vi "Read_LogFiles (Host Computer).vi"() -> ()   [LabVIEW 2017]
uses:
  <vilib>/Utility/file.llb/Read From Spreadsheet File (DBL).vi
panel:
  out "Graph 3":cluster{dbl[], dbl[]}(graph)
  out "Graph 2":cluster{"Y":dbl[], "Y":dbl[]}[](graph)
  out "Graph 1":cluster{"Y":dbl[], "Y":dbl[]}[](graph)
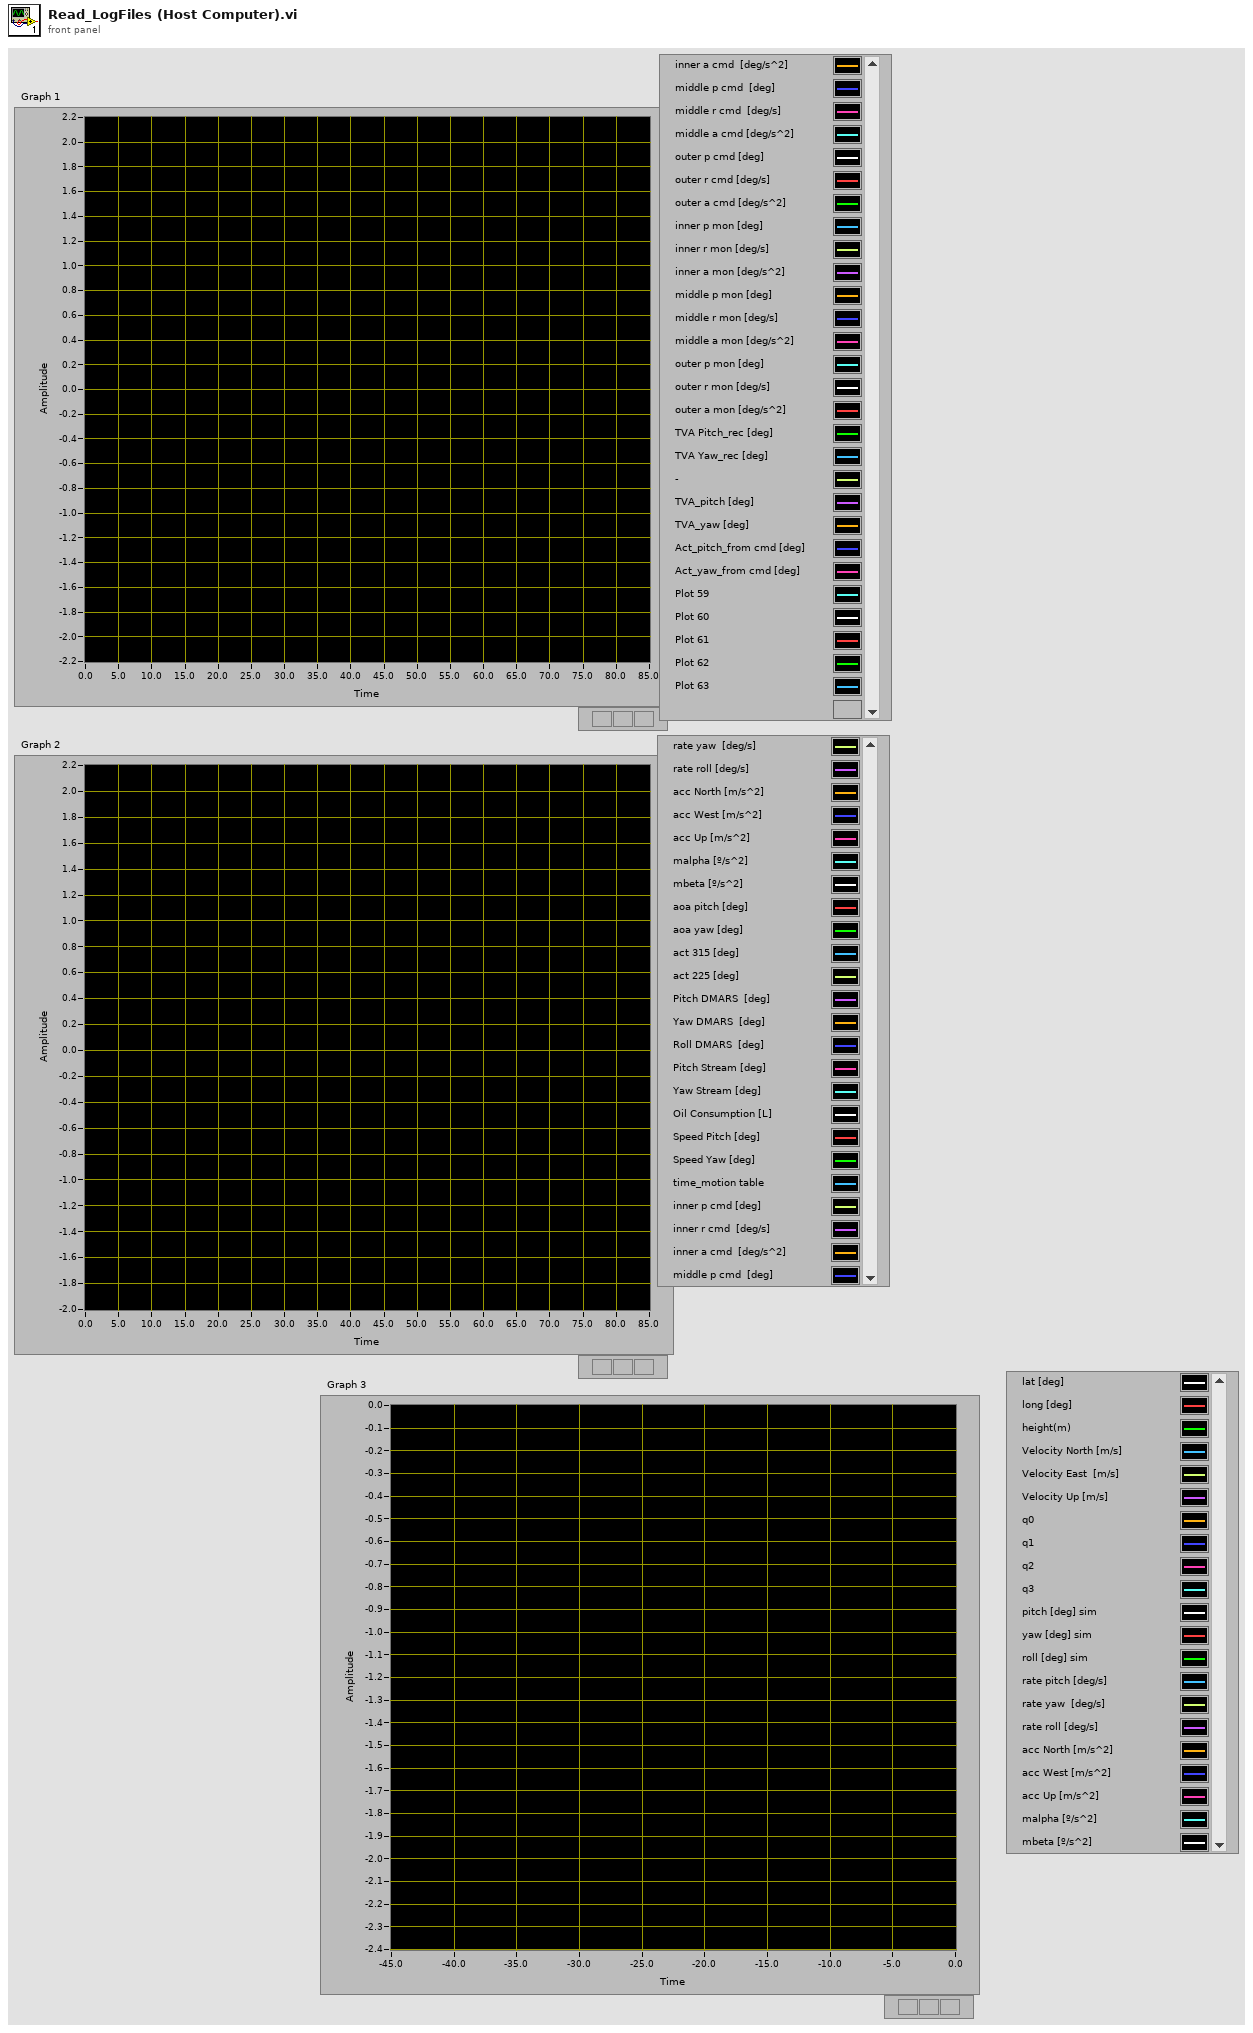
[diagram p1: front panel]
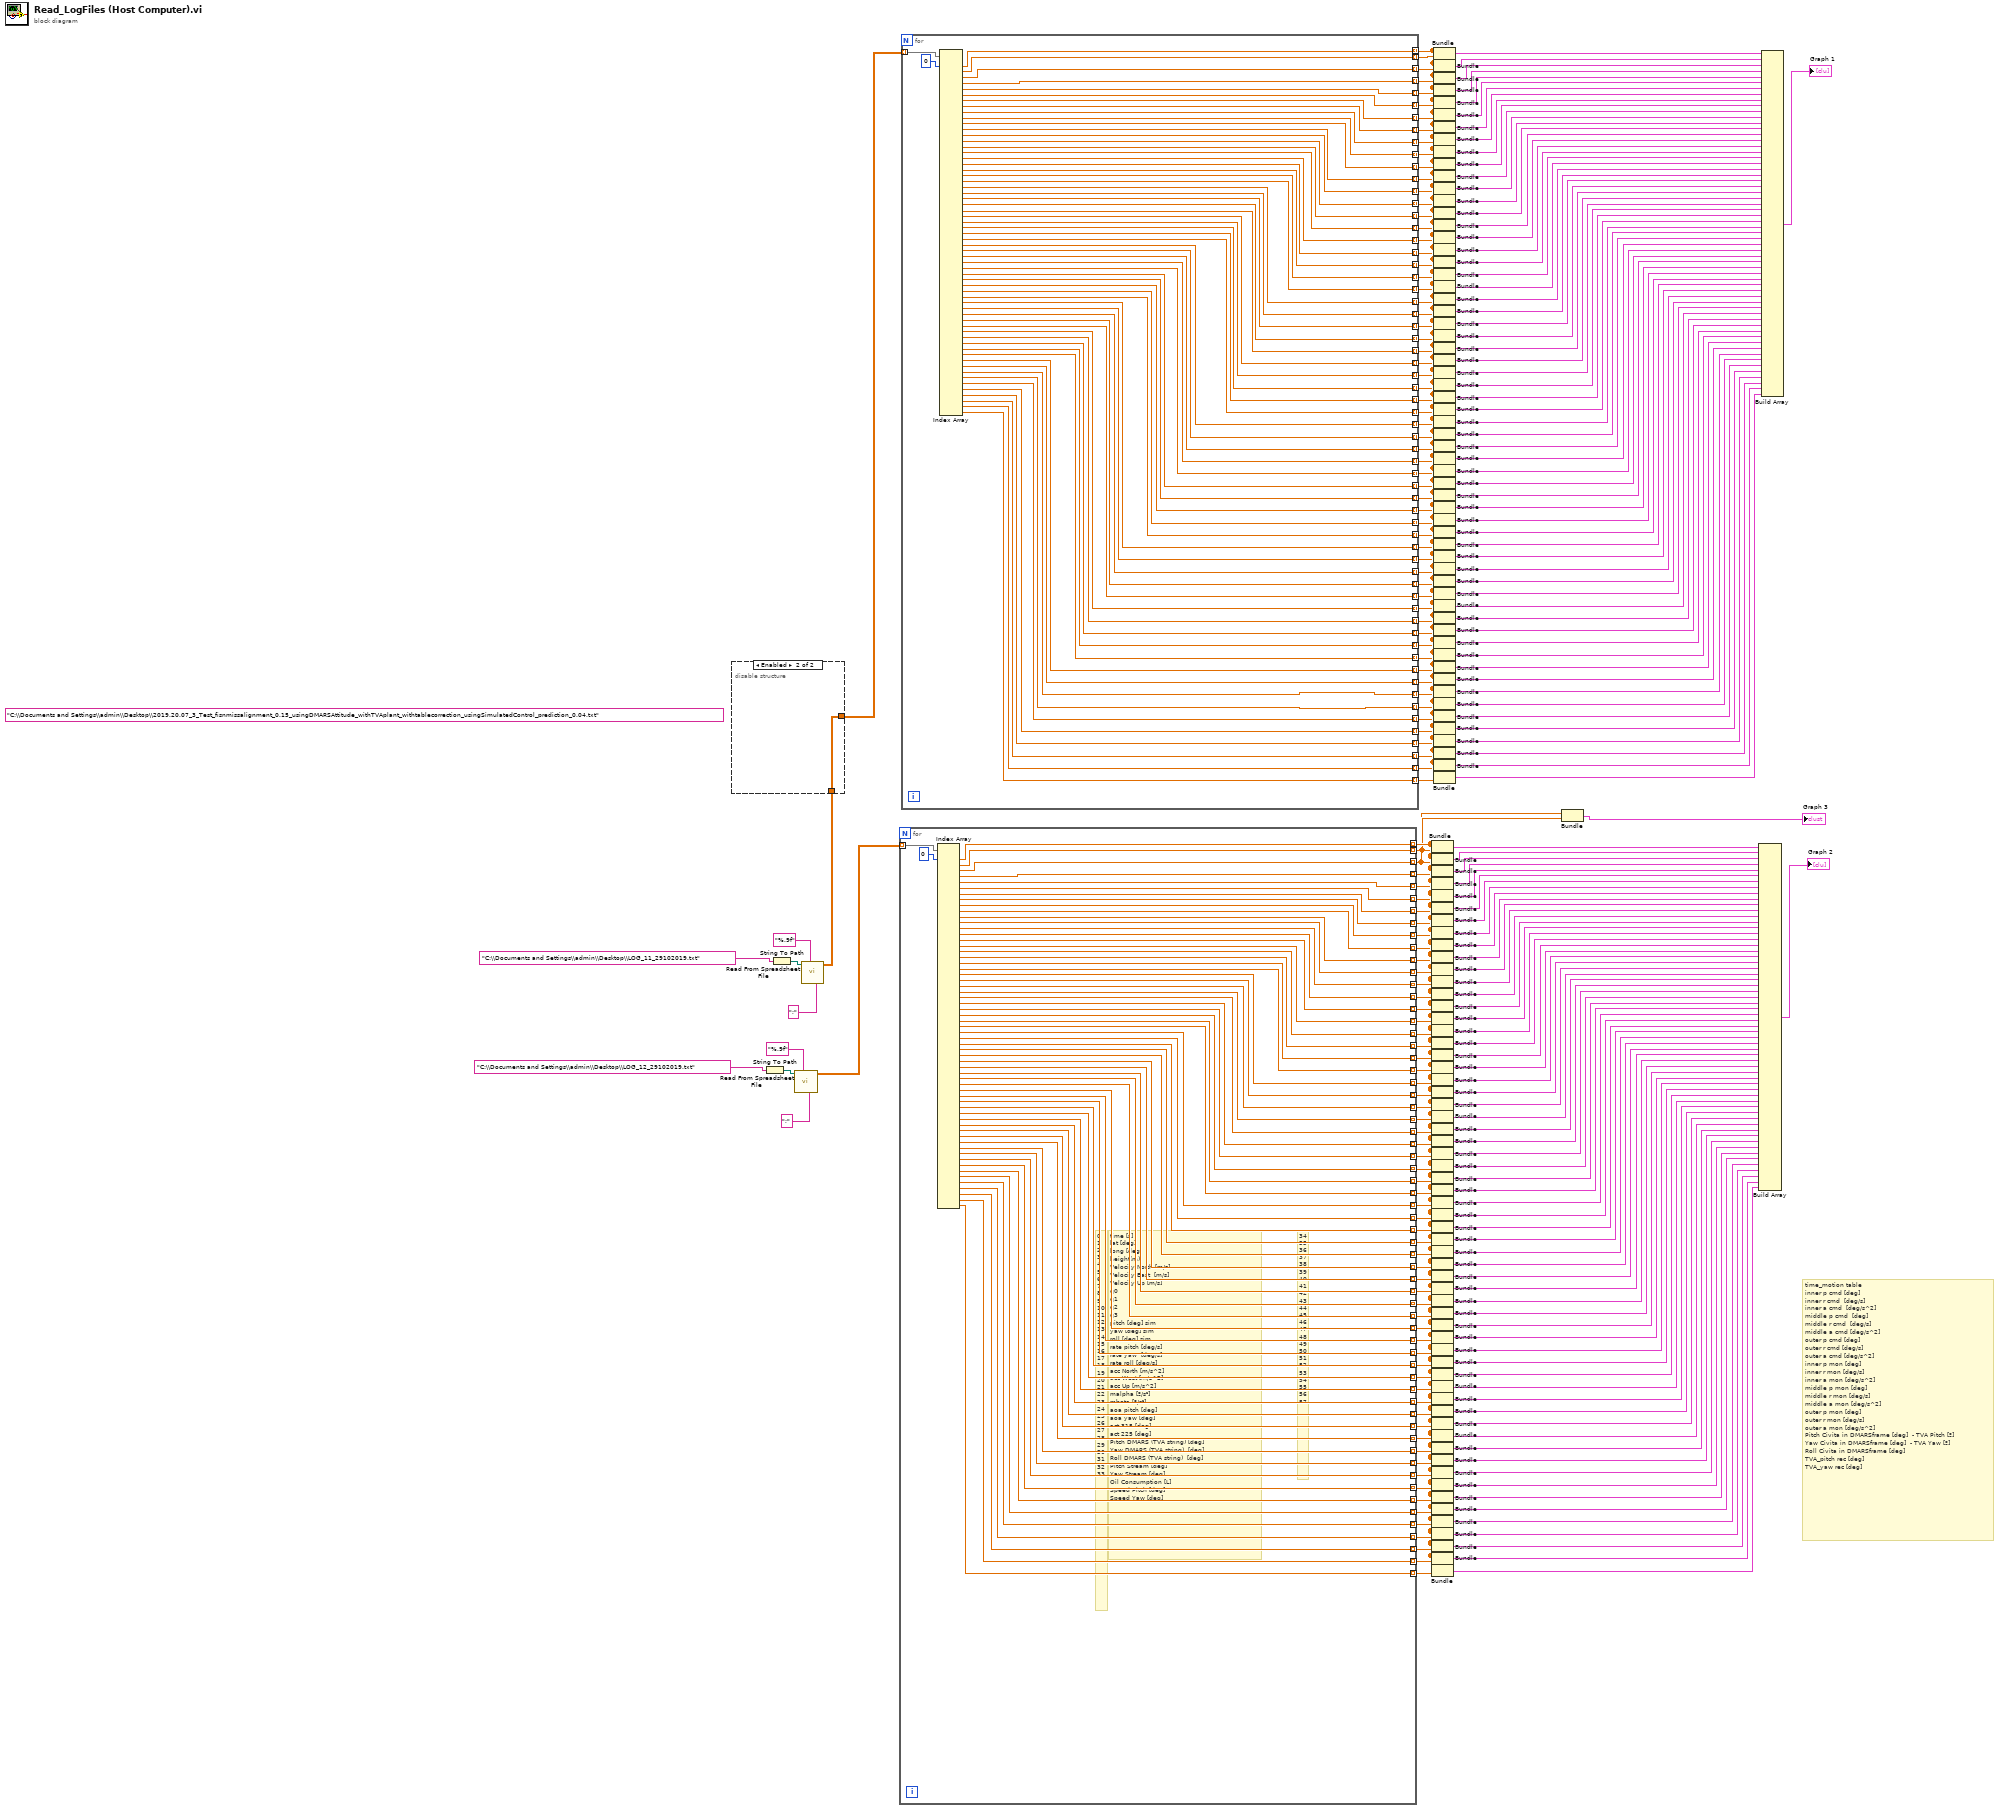
[diagram p0: block diagram]
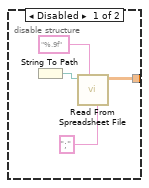
[diagram p2: hidden frame]
diagram:
  (unwired) "C:\\Documents and Settings\\admin\\Desktop\\2019.20.07_3_Test_fisnmissalignment_0.15_usingDMARSAttitude_withTVAplant_withtablecorrection_usingSimulatedControl_prediction_0.04.txt" ("format (%.3f)")
  # "time_motion table\ninner p cmd [deg]\ninner r cmd  [deg/s]\ninner a cmd  [deg/s^2]\nmiddle p cmd  [deg]\nmiddle r cmd  [deg/s]\nmiddle a cmd [deg/s^2]\nouter p cmd [deg]\nouter r cmd [deg/s]\nouter a cmd [deg/s^2]\ninner p mon [deg]\ninner r mon [deg/s]\ninner a mon [deg/s^2]\nmiddle p mon [deg]\nmiddle r mon [deg/s]\nmiddle a mon [deg/s^2]\nouter p mon [deg]\nouter r mon [deg/s]\nouter a mon [deg/s^2]\nPitch Civita in DMARSframe [deg]  - TVA Pitch [º]\nYaw Civita in DMARSframe [deg]  - TVA Yaw [º]\nRoll Civita in DMARSframe [deg]\nTVA_pitch rec [deg]\nTVA_yaw rec [deg]"
  # "34\n35\n36\n37\n38\n39\n40\n41\n42\n43\n44\n45\n46\n47\n48\n49\n50\n51\n52\n53\n54\n55\n56\n57"
  # "0\n1\n2\n3\n4\n5\n6\n7\n8\n9\n10\n11\n12\n13\n14\n15\n16\n17\n18\n19\n20\n21\n22\n23\n24\n25\n26\n27\n28\n29\n30\n31\n32\n33"
  # "time [s]\nlat [deg]\nlong [deg]\nheight(m)\nVelocity North [m/s]\nVelocity East  [m/s]\nVelocity Up [m/s]\nq0\nq1\nq2\nq3\npitch [deg] sim\nyaw [deg] sim\nroll [deg] sim\nrate pitch [deg/s] \nrate yaw  [deg/s]\nrate roll [deg/s]\nacc North [m/s^2] \nacc West [m/s^2]\nacc Up [m/s^2]\nmalpha [º/s²]\nmbeta [º/s²]\naoa pitch [deg] \naoa yaw [deg]\nact 315 [deg] \nact 225 [deg]\nPitch DMARS (TVA string) [deg]\nYaw DMARS (TVA string)  [deg]\nRoll DMARS (TVA string)  [deg]\nPitch Stream [deg]\nYaw Stream [deg]\nOil Consumption [L]\nSpeed Pitch [deg]\nSpeed Yaw [deg]"
  n1 = String To Path(string="C:\\Documents and Settings\\admin\\Desktop\\LOG_12_29102019.txt" ("format (%.3f)")) -> (path=w127:path)
  n2 = String To Path(string="C:\\Documents and Settings\\admin\\Desktop\\LOG_11_29102019.txt" ("format (%.3f)")) -> (path=w254:path)
  n3 = call-poly <vilib>:"Read From Spreadsheet File.vi"("delimiter (\\t)"=";" ("delimiter (\\t)"), "format (%.3f)"="%.9f", "file path (dialog if empty)"=w127) -> ("all rows"=w4:dbl[][])  [unwired: 4 in, 4 out]
  n4 = call-poly <vilib>:"Read From Spreadsheet File.vi"("delimiter (\\t)"=";" ("delimiter (\\t)"), "format (%.3f)"="%.9f", "file path (dialog if empty)"=w254) -> ("all rows"=w252:dbl[][])  [unwired: 4 in, 4 out]
  n5 = disable-structure shown="Enabled" {
    disable-tunnel: [w260 w261] -> w251
    disable-tunnel: w252 -> [_ w261]
    frame Disabled {
      n6 = String To Path() -> (path=w259:path)  [unwired: 1 in]
      n7 = call-poly <vilib>:"Read From Spreadsheet File.vi"("delimiter (\\t)"=";" ("delimiter (\\t)"), "format (%.3f)"="%.9f", "file path (dialog if empty)"=w259) -> ("all rows"=w260:dbl[][])  [unwired: 4 in, 4 out]
    }
    frame Enabled {
    }
  }
  n8 = for {
    tunnel: w4 -> [w264] mode=indexing
    tunnel: [w323] -> w24 mode=indexing
    tunnel: [w320] -> w3 mode=indexing
    tunnel: [w319] -> w2 mode=indexing
    tunnel: [w321] -> w12 mode=indexing
    tunnel: [w318] -> w10 mode=indexing
    tunnel: [w322] -> w8 mode=indexing
    tunnel: [w266] -> w7 mode=indexing
    tunnel: [w317] -> w16 mode=indexing
    tunnel: [w316] -> w21 mode=indexing
    tunnel: [w315] -> w22 mode=indexing
    tunnel: [w314] -> w23 mode=indexing
    tunnel: [w313] -> w25 mode=indexing
    tunnel: [w312] -> w26 mode=indexing
    tunnel: [w311] -> w27 mode=indexing
    tunnel: [w310] -> w28 mode=indexing
    tunnel: [w309] -> w29 mode=indexing
    tunnel: [w308] -> w30 mode=indexing
    tunnel: [w307] -> w31 mode=indexing
    tunnel: [w306] -> w32 mode=indexing
    tunnel: [w305] -> w33 mode=indexing
    tunnel: [w304] -> w34 mode=indexing
    tunnel: [w303] -> w35 mode=indexing
    tunnel: [w302] -> w36 mode=indexing
    tunnel: [w301] -> w37 mode=indexing
    tunnel: [w267] -> w38 mode=indexing
    tunnel: [w300] -> w39 mode=indexing
    tunnel: [w299] -> w40 mode=indexing
    tunnel: [w298] -> w41 mode=indexing
    tunnel: [w297] -> w42 mode=indexing
    tunnel: [w296] -> w43 mode=indexing
    tunnel: [w295] -> w44 mode=indexing
    tunnel: [w294] -> w45 mode=indexing
    tunnel: [w293] -> w46 mode=indexing
    tunnel: [w292] -> w47 mode=indexing
    tunnel: [w291] -> w48 mode=indexing
    tunnel: [w290] -> w49 mode=indexing
    tunnel: [w289] -> w50 mode=indexing
    tunnel: [w288] -> w51 mode=indexing
    tunnel: [w287] -> w52 mode=indexing
    tunnel: [w265] -> w53 mode=indexing
    tunnel: [w286] -> w54 mode=indexing
    tunnel: [w285] -> w55 mode=indexing
    tunnel: [w284] -> w56 mode=indexing
    tunnel: [w283] -> w57 mode=indexing
    tunnel: [w282] -> w58 mode=indexing
    tunnel: [w281] -> w59 mode=indexing
    tunnel: [w280] -> w60 mode=indexing
    tunnel: [w279] -> w61 mode=indexing
    tunnel: [w278] -> w62 mode=indexing
    tunnel: [w277] -> w63 mode=indexing
    tunnel: [w276] -> w64 mode=indexing
    tunnel: [w275] -> w65 mode=indexing
    tunnel: [w274] -> w66 mode=indexing
    tunnel: [w273] -> w67 mode=indexing
    tunnel: [w272] -> w68 mode=indexing
    tunnel: [w271] -> w69 mode=indexing
    tunnel: [w270] -> w70 mode=indexing
    tunnel: [w269] -> w71 mode=indexing
    tunnel: [w268] -> w72 mode=indexing
    tunnel: [w263] -> w73 mode=indexing
    tunnel: [w262] -> w74 mode=indexing
    n9 = Index Array(array=w264, index #1=0 ("index")) -> (element #1=w323:dbl, element #2=w320:dbl, element #3=w319:dbl, element #4=w321:dbl, element #5=w318:dbl, element #6=w317:dbl, element #7=w316:dbl, element #8=w315:dbl, element #9=w314:dbl, element #10=w322:dbl, element #11=w266:dbl, element #12=w313:dbl, element #13=w312:dbl, element #14=w311:dbl, element #15=w310:dbl, element #16=w309:dbl, element #17=w308:dbl, element #18=w307:dbl, element #19=w306:dbl, element #20=w305:dbl, element #21=w304:dbl, element #22=w303:dbl, element #23=w302:dbl, element #24=w301:dbl, element #25=w267:dbl, element #26=w300:dbl, element #27=w299:dbl, element #28=w298:dbl, element #29=w297:dbl, element #30=w296:dbl, element #31=w295:dbl, element #32=w294:dbl, element #33=w293:dbl, element #34=w292:dbl, element #35=w291:dbl, element #36=w290:dbl, element #37=w289:dbl, element #38=w288:dbl, element #39=w287:dbl, element #40=w265:dbl, element #41=w286:dbl, element #42=w285:dbl, element #43=w284:dbl, element #44=w283:dbl, element #45=w282:dbl, element #46=w281:dbl, element #47=w280:dbl, element #48=w279:dbl, element #49=w278:dbl, element #50=w277:dbl, element #51=w276:dbl, element #52=w275:dbl, element #53=w274:dbl, element #54=w273:dbl, element #55=w272:dbl, element #56=w271:dbl, element #57=w270:dbl, element #58=w269:dbl, element #59=w268:dbl, element #60=w263:dbl, element #61=w262:dbl)  [unwired: 60 in]
  }
  n10 = for {
    tunnel: w251 -> [w387] mode=indexing
    tunnel: [w385] -> w229 mode=indexing
    tunnel: [w381] -> w241 mode=indexing
    tunnel: [w380] -> w242 mode=indexing
    tunnel: [w382] -> w243 mode=indexing
    tunnel: [w379] -> w245 mode=indexing
    tunnel: [w384] -> w247 mode=indexing
    tunnel: [w383] -> w248 mode=indexing
    tunnel: [w378] -> w237 mode=indexing
    tunnel: [w377] -> w232 mode=indexing
    tunnel: [w376] -> w231 mode=indexing
    tunnel: [w375] -> w230 mode=indexing
    tunnel: [w374] -> w228 mode=indexing
    tunnel: [w373] -> w227 mode=indexing
    tunnel: [w372] -> w226 mode=indexing
    tunnel: [w371] -> w225 mode=indexing
    tunnel: [w370] -> w224 mode=indexing
    tunnel: [w369] -> w223 mode=indexing
    tunnel: [w368] -> w222 mode=indexing
    tunnel: [w367] -> w221 mode=indexing
    tunnel: [w366] -> w220 mode=indexing
    tunnel: [w365] -> w219 mode=indexing
    tunnel: [w364] -> w218 mode=indexing
    tunnel: [w363] -> w217 mode=indexing
    tunnel: [w329] -> w216 mode=indexing
    tunnel: [w325] -> w215 mode=indexing
    tunnel: [w326] -> w214 mode=indexing
    tunnel: [w362] -> w213 mode=indexing
    tunnel: [w361] -> w212 mode=indexing
    tunnel: [w360] -> w211 mode=indexing
    tunnel: [w359] -> w210 mode=indexing
    tunnel: [w358] -> w209 mode=indexing
    tunnel: [w357] -> w208 mode=indexing
    tunnel: [w356] -> w207 mode=indexing
    tunnel: [w355] -> w206 mode=indexing
    tunnel: [w354] -> w205 mode=indexing
    tunnel: [w353] -> w204 mode=indexing
    tunnel: [w352] -> w203 mode=indexing
    tunnel: [w351] -> w202 mode=indexing
    tunnel: [w350] -> w201 mode=indexing
    tunnel: [w349] -> w200 mode=indexing
    tunnel: [w348] -> w199 mode=indexing
    tunnel: [w347] -> w198 mode=indexing
    tunnel: [w346] -> w197 mode=indexing
    tunnel: [w345] -> w196 mode=indexing
    tunnel: [w344] -> w195 mode=indexing
    tunnel: [w343] -> w194 mode=indexing
    tunnel: [w342] -> w193 mode=indexing
    tunnel: [w341] -> w192 mode=indexing
    tunnel: [w340] -> w191 mode=indexing
    tunnel: [w339] -> w190 mode=indexing
    tunnel: [w338] -> w189 mode=indexing
    tunnel: [w337] -> w188 mode=indexing
    tunnel: [w336] -> w187 mode=indexing
    tunnel: [w328] -> w186 mode=indexing
    tunnel: [w327] -> w185 mode=indexing
    tunnel: [w335] -> w184 mode=indexing
    tunnel: [w334] -> w183 mode=indexing
    tunnel: [w333] -> w182 mode=indexing
    tunnel: [w332] -> w181 mode=indexing
    tunnel: [w331] -> w180 mode=indexing
    tunnel: [w330] -> w179 mode=indexing
    n11 = Index Array(array=w387, index #1=0 ("index")) -> (element #1=w385:dbl, element #2=w381:dbl, element #3=w380:dbl, element #4=w382:dbl, element #5=w379:dbl, element #6=w378:dbl, element #7=w377:dbl, element #8=w376:dbl, element #9=w375:dbl, element #10=w384:dbl, element #11=w383:dbl, element #12=w374:dbl, element #13=w373:dbl, element #14=w372:dbl, element #15=w371:dbl, element #16=w370:dbl, element #17=w369:dbl, element #18=w368:dbl, element #19=w367:dbl, element #20=w366:dbl, element #21=w365:dbl, element #22=w364:dbl, element #23=w363:dbl, element #24=w329:dbl, element #25=w325:dbl, element #26=w326:dbl, element #27=w362:dbl, element #28=w361:dbl, element #29=w360:dbl, element #30=w359:dbl, element #31=w358:dbl, element #32=w357:dbl, element #33=w356:dbl, element #34=w355:dbl, element #35=w354:dbl, element #36=w353:dbl, element #37=w352:dbl, element #38=w351:dbl, element #39=w350:dbl, element #40=w349:dbl, element #41=w348:dbl, element #42=w347:dbl, element #43=w346:dbl, element #44=w345:dbl, element #45=w344:dbl, element #46=w343:dbl, element #47=w342:dbl, element #48=w341:dbl, element #49=w340:dbl, element #50=w339:dbl, element #51=w338:dbl, element #52=w337:dbl, element #53=w336:dbl, element #54=w328:dbl, element #55=w327:dbl, element #56=w335:dbl, element #57=w334:dbl, element #58=w333:dbl, element #59=w332:dbl, element #60=w331:dbl, element #61=w330:dbl)  [unwired: 60 in]
  }
  n12 = Bundle(w24, w3) -> (w15:cluster{dbl[], dbl[]})  [unwired: 1 in]
  n13 = Bundle(w24, w2) -> (w14:cluster{dbl[], dbl[]})  [unwired: 1 in]
  n14 = Bundle(w24, w12) -> (w11:cluster{dbl[], dbl[]})  [unwired: 1 in]
  n15 = Bundle(w24, w10) -> (w9:cluster{dbl[], dbl[]})  [unwired: 1 in]
  n16 = Bundle(w24, w16) -> (w17:cluster{dbl[], dbl[]})  [unwired: 1 in]
  n17 = Bundle(w24, w21) -> (w20:cluster{dbl[], dbl[]})  [unwired: 1 in]
  n18 = Bundle(w24, w22) -> (w19:cluster{dbl[], dbl[]})  [unwired: 1 in]
  n19 = Bundle(w24, w23) -> (w18:cluster{dbl[], dbl[]})  [unwired: 1 in]
  n20 = Bundle(w24, w8) -> (w6:cluster{dbl[], dbl[]})  [unwired: 1 in]
  n21 = Bundle(w24, w7) -> (w5:cluster{dbl[], dbl[]})  [unwired: 1 in]
  n22 = Bundle(w24, w25) -> (w75:cluster{dbl[], dbl[]})  [unwired: 1 in]
  n23 = Bundle(w24, w26) -> (w76:cluster{dbl[], dbl[]})  [unwired: 1 in]
  n24 = Bundle(w24, w27) -> (w77:cluster{dbl[], dbl[]})  [unwired: 1 in]
  n25 = Bundle(w24, w28) -> (w78:cluster{dbl[], dbl[]})  [unwired: 1 in]
  n26 = Bundle(w24, w29) -> (w79:cluster{dbl[], dbl[]})  [unwired: 1 in]
  n27 = Bundle(w24, w30) -> (w80:cluster{dbl[], dbl[]})  [unwired: 1 in]
  n28 = Bundle(w24, w31) -> (w81:cluster{dbl[], dbl[]})  [unwired: 1 in]
  n29 = Bundle(w24, w32) -> (w82:cluster{dbl[], dbl[]})  [unwired: 1 in]
  n30 = Bundle(w24, w33) -> (w83:cluster{dbl[], dbl[]})  [unwired: 1 in]
  n31 = Bundle(w24, w34) -> (w84:cluster{dbl[], dbl[]})  [unwired: 1 in]
  n32 = Bundle(w24, w35) -> (w85:cluster{dbl[], dbl[]})  [unwired: 1 in]
  n33 = Bundle(w24, w36) -> (w86:cluster{dbl[], dbl[]})  [unwired: 1 in]
  n34 = Bundle(w24, w37) -> (w87:cluster{dbl[], dbl[]})  [unwired: 1 in]
  n35 = Bundle(w24, w38) -> (w88:cluster{dbl[], dbl[]})  [unwired: 1 in]
  n36 = Bundle(w24, w39) -> (w89:cluster{dbl[], dbl[]})  [unwired: 1 in]
  n37 = Bundle(w24, w40) -> (w90:cluster{dbl[], dbl[]})  [unwired: 1 in]
  n38 = Bundle(w24, w41) -> (w91:cluster{dbl[], dbl[]})  [unwired: 1 in]
  n39 = Bundle(w24, w42) -> (w92:cluster{dbl[], dbl[]})  [unwired: 1 in]
  n40 = Bundle(w24, w43) -> (w93:cluster{dbl[], dbl[]})  [unwired: 1 in]
  n41 = Bundle(w24, w44) -> (w94:cluster{dbl[], dbl[]})  [unwired: 1 in]
  n42 = Bundle(w24, w45) -> (w95:cluster{dbl[], dbl[]})  [unwired: 1 in]
  n43 = Bundle(w24, w46) -> (w96:cluster{dbl[], dbl[]})  [unwired: 1 in]
  n44 = Bundle(w24, w47) -> (w97:cluster{dbl[], dbl[]})  [unwired: 1 in]
  n45 = Bundle(w24, w48) -> (w98:cluster{dbl[], dbl[]})  [unwired: 1 in]
  n46 = Bundle(w24, w49) -> (w99:cluster{dbl[], dbl[]})  [unwired: 1 in]
  n47 = Bundle(w24, w50) -> (w100:cluster{dbl[], dbl[]})  [unwired: 1 in]
  n48 = Bundle(w24, w51) -> (w101:cluster{dbl[], dbl[]})  [unwired: 1 in]
  n49 = Bundle(w24, w52) -> (w102:cluster{dbl[], dbl[]})  [unwired: 1 in]
  n50 = Bundle(w24, w53) -> (w103:cluster{dbl[], dbl[]})  [unwired: 1 in]
  n51 = Bundle(w24, w54) -> (w104:cluster{dbl[], dbl[]})  [unwired: 1 in]
  n52 = Bundle(w24, w55) -> (w105:cluster{dbl[], dbl[]})  [unwired: 1 in]
  n53 = Bundle(w24, w56) -> (w106:cluster{dbl[], dbl[]})  [unwired: 1 in]
  n54 = Bundle(w24, w57) -> (w107:cluster{dbl[], dbl[]})  [unwired: 1 in]
  n55 = Bundle(w24, w58) -> (w108:cluster{dbl[], dbl[]})  [unwired: 1 in]
  n56 = Bundle(w24, w59) -> (w109:cluster{dbl[], dbl[]})  [unwired: 1 in]
  n57 = Bundle(w24, w60) -> (w110:cluster{dbl[], dbl[]})  [unwired: 1 in]
  n58 = Bundle(w24, w61) -> (w111:cluster{dbl[], dbl[]})  [unwired: 1 in]
  n59 = Bundle(w24, w62) -> (w112:cluster{dbl[], dbl[]})  [unwired: 1 in]
  n60 = Bundle(w24, w63) -> (w113:cluster{dbl[], dbl[]})  [unwired: 1 in]
  n61 = Bundle(w24, w64) -> (w114:cluster{dbl[], dbl[]})  [unwired: 1 in]
  n62 = Bundle(w24, w65) -> (w115:cluster{dbl[], dbl[]})  [unwired: 1 in]
  n63 = Bundle(w24, w66) -> (w116:cluster{dbl[], dbl[]})  [unwired: 1 in]
  n64 = Bundle(w24, w67) -> (w117:cluster{dbl[], dbl[]})  [unwired: 1 in]
  n65 = Bundle(w24, w68) -> (w118:cluster{dbl[], dbl[]})  [unwired: 1 in]
  n66 = Bundle(w24, w69) -> (w119:cluster{dbl[], dbl[]})  [unwired: 1 in]
  n67 = Bundle(w24, w70) -> (w120:cluster{dbl[], dbl[]})  [unwired: 1 in]
  n68 = Bundle(w24, w71) -> (w121:cluster{dbl[], dbl[]})  [unwired: 1 in]
  n69 = Bundle(w24, w72) -> (w122:cluster{dbl[], dbl[]})  [unwired: 1 in]
  n70 = Bundle(w24, w73) -> (w123:cluster{dbl[], dbl[]})  [unwired: 1 in]
  n71 = Bundle(w24, w74) -> (w124:cluster{dbl[], dbl[]})  [unwired: 1 in]
  n72 = Bundle(w229, w241) -> (w238:cluster{dbl[], dbl[]})  [unwired: 1 in]
  n73 = Bundle(w229, w242) -> (w239:cluster{dbl[], dbl[]})  [unwired: 1 in]
  n74 = Bundle(w229, w243) -> (w244:cluster{dbl[], dbl[]})  [unwired: 1 in]
  n75 = Bundle(w229, w245) -> (w246:cluster{dbl[], dbl[]})  [unwired: 1 in]
  n76 = Bundle(w229, w237) -> (w236:cluster{dbl[], dbl[]})  [unwired: 1 in]
  n77 = Bundle(w229, w232) -> (w233:cluster{dbl[], dbl[]})  [unwired: 1 in]
  n78 = Bundle(w229, w231) -> (w234:cluster{dbl[], dbl[]})  [unwired: 1 in]
  n79 = Bundle(w229, w230) -> (w235:cluster{dbl[], dbl[]})  [unwired: 1 in]
  n80 = Bundle(w229, w247) -> (w249:cluster{dbl[], dbl[]})  [unwired: 1 in]
  n81 = Bundle(w229, w248) -> (w250:cluster{dbl[], dbl[]})  [unwired: 1 in]
  n82 = Bundle(w229, w228) -> (w178:cluster{dbl[], dbl[]})  [unwired: 1 in]
  n83 = Bundle(w229, w227) -> (w177:cluster{dbl[], dbl[]})  [unwired: 1 in]
  n84 = Bundle(w229, w226) -> (w176:cluster{dbl[], dbl[]})  [unwired: 1 in]
  n85 = Bundle(w229, w225) -> (w175:cluster{dbl[], dbl[]})  [unwired: 1 in]
  n86 = Bundle(w229, w224) -> (w174:cluster{dbl[], dbl[]})  [unwired: 1 in]
  n87 = Bundle(w229, w223) -> (w173:cluster{dbl[], dbl[]})  [unwired: 1 in]
  n88 = Bundle(w229, w222) -> (w172:cluster{dbl[], dbl[]})  [unwired: 1 in]
  n89 = Bundle(w229, w221) -> (w171:cluster{dbl[], dbl[]})  [unwired: 1 in]
  n90 = Bundle(w229, w220) -> (w170:cluster{dbl[], dbl[]})  [unwired: 1 in]
  n91 = Bundle(w229, w219) -> (w169:cluster{dbl[], dbl[]})  [unwired: 1 in]
  n92 = Bundle(w229, w218) -> (w168:cluster{dbl[], dbl[]})  [unwired: 1 in]
  n93 = Bundle(w229, w217) -> (w167:cluster{dbl[], dbl[]})  [unwired: 1 in]
  n94 = Bundle(w229, w216) -> (w166:cluster{dbl[], dbl[]})  [unwired: 1 in]
  n95 = Bundle(w229, w215) -> (w165:cluster{dbl[], dbl[]})  [unwired: 1 in]
  n96 = Bundle(w229, w214) -> (w164:cluster{dbl[], dbl[]})  [unwired: 1 in]
  n97 = Bundle(w229, w213) -> (w163:cluster{dbl[], dbl[]})  [unwired: 1 in]
  n98 = Bundle(w229, w212) -> (w162:cluster{dbl[], dbl[]})  [unwired: 1 in]
  n99 = Bundle(w229, w211) -> (w161:cluster{dbl[], dbl[]})  [unwired: 1 in]
  n100 = Bundle(w229, w210) -> (w160:cluster{dbl[], dbl[]})  [unwired: 1 in]
  n101 = Bundle(w229, w209) -> (w159:cluster{dbl[], dbl[]})  [unwired: 1 in]
  n102 = Bundle(w229, w208) -> (w158:cluster{dbl[], dbl[]})  [unwired: 1 in]
  n103 = Bundle(w229, w207) -> (w157:cluster{dbl[], dbl[]})  [unwired: 1 in]
  n104 = Bundle(w229, w206) -> (w156:cluster{dbl[], dbl[]})  [unwired: 1 in]
  n105 = Bundle(w229, w205) -> (w155:cluster{dbl[], dbl[]})  [unwired: 1 in]
  n106 = Bundle(w229, w204) -> (w154:cluster{dbl[], dbl[]})  [unwired: 1 in]
  n107 = Bundle(w229, w203) -> (w153:cluster{dbl[], dbl[]})  [unwired: 1 in]
  n108 = Bundle(w229, w202) -> (w152:cluster{dbl[], dbl[]})  [unwired: 1 in]
  n109 = Bundle(w229, w201) -> (w151:cluster{dbl[], dbl[]})  [unwired: 1 in]
  n110 = Bundle(w229, w200) -> (w150:cluster{dbl[], dbl[]})  [unwired: 1 in]
  n111 = Bundle(w229, w199) -> (w149:cluster{dbl[], dbl[]})  [unwired: 1 in]
  n112 = Bundle(w229, w198) -> (w148:cluster{dbl[], dbl[]})  [unwired: 1 in]
  n113 = Bundle(w229, w197) -> (w147:cluster{dbl[], dbl[]})  [unwired: 1 in]
  n114 = Bundle(w229, w196) -> (w146:cluster{dbl[], dbl[]})  [unwired: 1 in]
  n115 = Bundle(w229, w195) -> (w145:cluster{dbl[], dbl[]})  [unwired: 1 in]
  n116 = Bundle(w229, w194) -> (w144:cluster{dbl[], dbl[]})  [unwired: 1 in]
  n117 = Bundle(w229, w193) -> (w143:cluster{dbl[], dbl[]})  [unwired: 1 in]
  n118 = Bundle(w229, w192) -> (w142:cluster{dbl[], dbl[]})  [unwired: 1 in]
  n119 = Bundle(w229, w191) -> (w141:cluster{dbl[], dbl[]})  [unwired: 1 in]
  n120 = Bundle(w229, w190) -> (w140:cluster{dbl[], dbl[]})  [unwired: 1 in]
  n121 = Bundle(w229, w189) -> (w139:cluster{dbl[], dbl[]})  [unwired: 1 in]
  n122 = Bundle(w229, w188) -> (w138:cluster{dbl[], dbl[]})  [unwired: 1 in]
  n123 = Bundle(w229, w187) -> (w137:cluster{dbl[], dbl[]})  [unwired: 1 in]
  n124 = Bundle(w229, w186) -> (w136:cluster{dbl[], dbl[]})  [unwired: 1 in]
  n125 = Bundle(w229, w185) -> (w135:cluster{dbl[], dbl[]})  [unwired: 1 in]
  n126 = Bundle(w229, w184) -> (w134:cluster{dbl[], dbl[]})  [unwired: 1 in]
  n127 = Bundle(w229, w183) -> (w133:cluster{dbl[], dbl[]})  [unwired: 1 in]
  n128 = Bundle(w229, w182) -> (w132:cluster{dbl[], dbl[]})  [unwired: 1 in]
  n129 = Bundle(w229, w181) -> (w131:cluster{dbl[], dbl[]})  [unwired: 1 in]
  n130 = Bundle(w229, w180) -> (w130:cluster{dbl[], dbl[]})  [unwired: 1 in]
  n131 = Bundle(w229, w179) -> (w129:cluster{dbl[], dbl[]})  [unwired: 1 in]
  n132 = Bundle(w2, w3) -> (→"Graph 3":cluster{dbl[], dbl[]})  [unwired: 1 in]
  n133 = Build Array(w15, w14, w11, w9, w17, w20, w19, w18, w6, w5, w75, w76, w77, w78, w79, w80, w81, w82, w83, w84, w85, w86, w87, w88, w89, w90, w91, w92, w93, w94, w95, w96, w97, w98, w99, w100, w101, w102, w103, w104, w105, w106, w107, w108, w109, w110, w111, w112, w113, w114, w115, w116, w117, w118, w119, w120, w121, w122, w123, w124) -> (→"Graph 2":cluster{dbl[], dbl[]}[])
  n134 = Build Array(w238, w239, w244, w246, w236, w233, w234, w235, w249, w250, w178, w177, w176, w175, w174, w173, w172, w171, w170, w169, w168, w167, w166, w165, w164, w163, w162, w161, w160, w159, w158, w157, w156, w155, w154, w153, w152, w151, w150, w149, w148, w147, w146, w145, w144, w143, w142, w141, w140, w139, w138, w137, w136, w135, w134, w133, w132, w131, w130, w129) -> (→"Graph 1":cluster{dbl[], dbl[]}[])
